vi "create.vi"(7 "ID":string, 9 "task token":refnum<class "null task token.lvclass">, 10 "results reporter":refnum<class "results reporter.lvclass">, 11 "action":refnum<class "action.lvclass">) -> (3 "function task out":refnum<class "function task.lvclass">)   [LabVIEW 2013, in "function task.lvclass"]
uses:
  function task.lvclass
  results reporter/results reporter.lvclass
  action/action.lvclass
  task token/null task token.lvclass
  function task.lvclass/function task.ctl
  task/task.lvclass/task.ctl
  task/task.lvclass
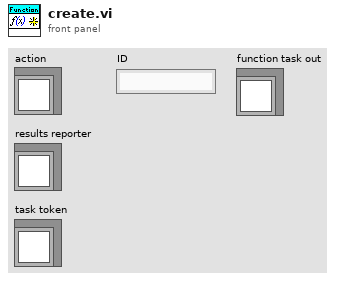
[diagram p1: front panel]
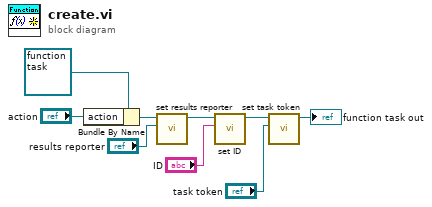
[diagram p0: block diagram]
diagram:
  n1 = Bundle By Name(cluster=refnum<class "function task.lvclass"> refnum ("function task in"), "action"="action") -> (w8:refnum<class "function task.lvclass">)
  n2 = call "set results reporter.vi"("results reporter"="results reporter", "task in"=w8) -> ("task out"=w7:refnum<class "function task.lvclass">)  [unwired: 9 in]
  n3 = call "set ID.vi"("ID"="ID", "task in"=w7) -> ("task out"=w4:refnum<class "function task.lvclass">)  [unwired: 9 in]
  n4 = call "set task token.vi"("task token"="task token", "task in"=w4) -> ("task out"=→"function task out":refnum<class "function task.lvclass">)  [unwired: 9 in]
